vi "Commit DAQ Tags.vi"(8 "error in (no error)":errorcluster, 11 "DAQ State in":T1) -> (0 "error out":errorcluster, 3 "DAQ State out":T1)   [LabVIEW 2018, in "DAQ.lvlib"]
uses:
  DAQ.lvlib
  Acquisition/Hardware Configuration.ctl
  Acquisition/Task Cluster.ctl
  Tag VIs/Tag FGV Operation Enum.ctl
  Shared Variables/Dynamic Shared Variables.lvlib
  <resource>/objmgr/daqmx.rc
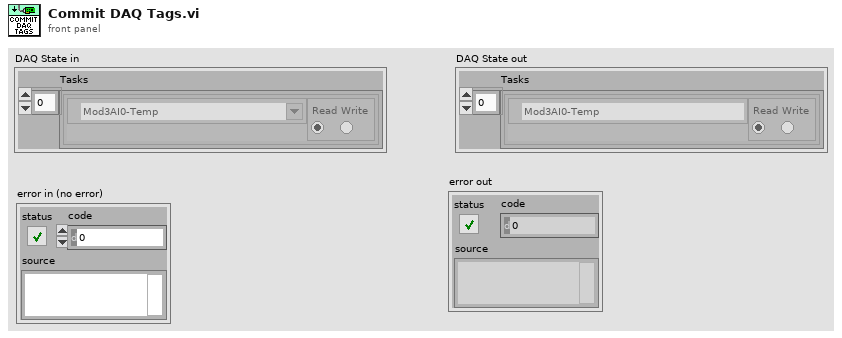
[diagram p1: front panel]
types:
  T1 = typedef "DAQ.lvlib/Hardware Configuration.ctl" = cluster{"Tasks":T2[]}
  T2 = typedef "Task Cluster.ctl" = cluster{"DAQmx Task":refnum<k21>, "Read-Write Radio":enum32{"Read", "Write"}}
  T3 = typedef "Tag FGV Operation Enum.ctl" = enum16{"Init", "Set Notification Queue", "Create Tag", "Commit", "Write Tag (Numeric)", "Write Tag (Boolean)", "Read All Tags", "Read One Tag", "Delete Tag Category", "Set Alarm Parameters (Numeric)", "Set Alarm Parameters (Boolean)", "Enable All Alarms", "Disable All Alarms", "Delete All Tags", "Read Alarms", "Ack Alarm"}
  T4 = enum32{"u32BitField", "bool", "double", "string", "int8", "uint8", "int16", "uint16", "int32", "uint32", "int64", "uint64", "single", "double waveform", "int16 waveform", "array of boolean", "array of int8", "array of uint8", "array of int16", "array of uint16", "array of int32", "array of uint32", "array of int64", "array of uint64", "array of single", "array of double", "array of double waveform", "array of int16 waveform", "array of string", "variant", "timestamp", "fixed point", "custom"}
  T5 = cluster{"enable? (F)":bool, "name":string, "alarm type":enum16{"HI_HI", "HI", "LO", "LO_LO"}, "level/change":dbl, "deadband/time":dbl, "priority":u32, "ack type":enum16{"Auto", "User", "None", "Each Occurrence"}, "area":string, "description":string, "log? (T)":bool}
  T6 = enum16{"Auto", "User", "None", "Each Occurrence"}
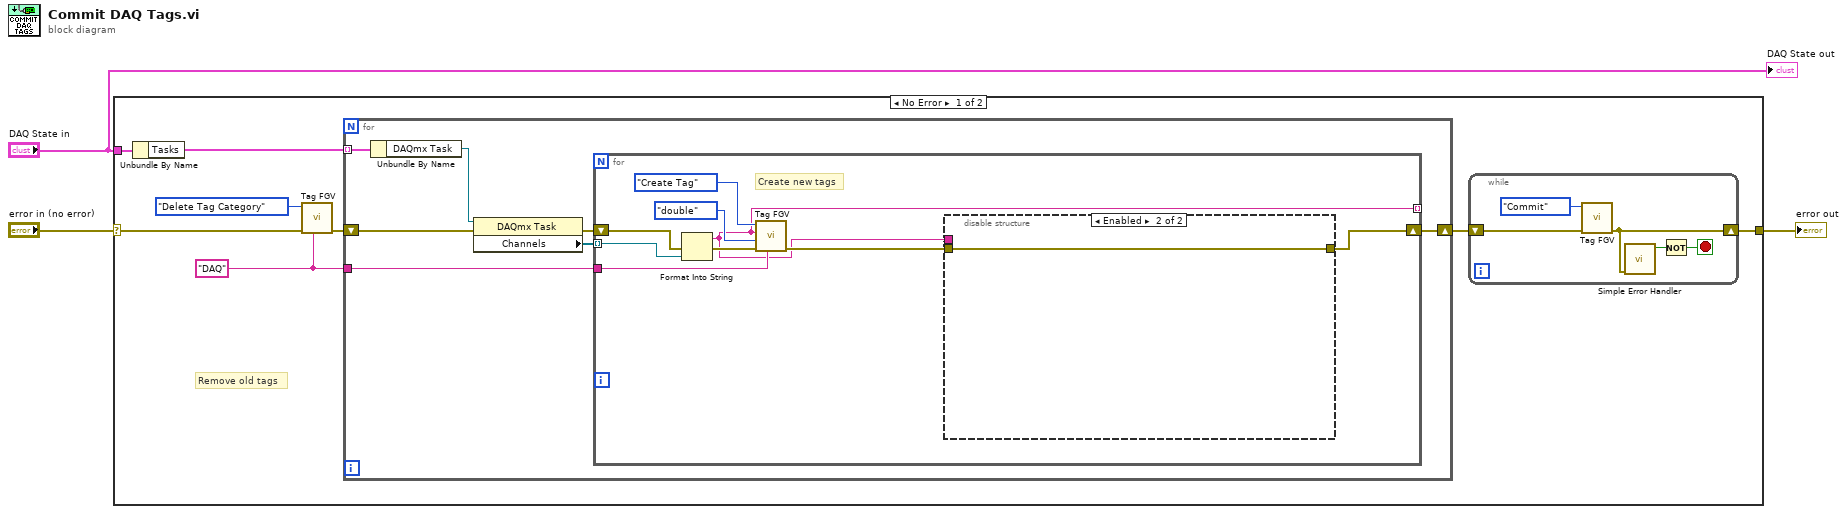
[diagram p0: block diagram]
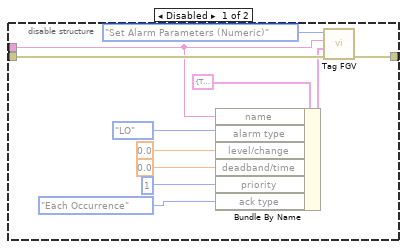
[diagram p2: hidden frame]
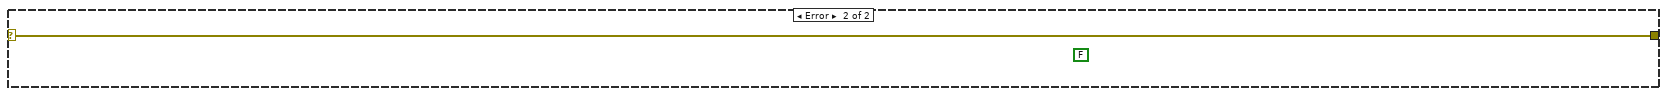
[diagram p3: hidden frame]
diagram:
  n1 = case shown="No Error" "error in (no error)" {
    selector: "error in (no error)" -> [w8 w45]
    tunnel: "DAQ State in" -> [w10 _]
    tunnel: [w4 w45] -> w1
    frame No Error {
      w6 = "DAQ" ("Tag Category")
      # "Remove old tags"
      n2 = Unbundle By Name(w10) -> ("Tasks"=w11:T2[])
      n3 = call "Tag FGV.vi"("Tag Category"=w6, "error in (no error)"=w8, "Operation"=Tag_FGV_Operation_Enum."Delete Tag Category") -> ("error out"=w7:errorcluster)  [unwired: 3 in, 5 out]
      n4 = for {
        tunnel: w11 -> [w23] mode=indexing
        shift-right: [w18] -> w5
        shift-left: w7 -> [w22]
        tunnel: w6 -> [w19]
        n5 = Unbundle By Name(w23) -> ("DAQmx Task"=w21:refnum<k21>)
        n6 = property class="DAQmx Task"(reference=w21, error in=w22) -> (error out=w17:errorcluster, "Channels"=w20:refnum<k21>[])  [unwired: 1 out]
        n7 = for {
          tunnel: w20 -> [w31] mode=indexing
          shift-right: [w25] -> w18
          shift-left: w17 -> [w30]
          tunnel: w19 -> [w27]
          tunnel: [w24] -> _ mode=indexing
          # "Create new tags"
          n8 = Format Into String(error in=w30, w31) -> (resulting string=w24:string, error out=w32:errorcluster)  [unwired: 2 in]
          n9 = call "Tag FGV.vi"("Tag Category"=w27, "error in (no error)"=w32, "Data"=T4."double" ("data type"), "Tag Name"=w24, "Operation"=Tag_FGV_Operation_Enum."Create Tag") -> ("error out"=w26:errorcluster)  [unwired: 1 in, 5 out]
          n10 = disable-structure shown="Enabled" {
            disable-tunnel: w26 -> [w42 w44]
            disable-tunnel: [w41 w44] -> w25
            disable-tunnel: w24 -> [w39 _]
            frame Disabled {
              n11 = Bundle By Name(cluster=T5 {"enable? (F)"=TRUE, "name"="HiHi", "alarm type"=enum."HI_HI", "level/change"=50.0, "deadband/time"=1.0, "priority"=1, "ack type"=enum."Each Occurrence", "area"="", "description"="", "log? (T)"=TRUE} ("numeric alarm settings"), "name"=w39, "alarm type"=enum16{"HI_HI", "HI", "LO", "LO_LO"}."LO", "level/change"=0.0, "deadband/time"=0.0, "priority"=u32 1, "ack type"=T6."Each Occurrence") -> (w33:T5)
              n12 = call "Tag FGV.vi"("error in (no error)"=w42, "Data"=w33, "Tag Name"=w39, "Operation"=Tag_FGV_Operation_Enum."Set Alarm Parameters (Numeric)") -> ("error out"=w41:errorcluster)  [unwired: 2 in, 5 out]
            }
            frame Enabled {
            }
          }
        }
      }
      n13 = while {
        shift-right: [w14] -> w4
        shift-left: w5 -> [w15]
        stop <- w12 stop-if-true
        n14 = call "Tag FGV.vi"("error in (no error)"=w15, "Operation"=Tag_FGV_Operation_Enum."Commit") -> ("error out"=w14:errorcluster)  [unwired: 4 in, 5 out]
        n15 = call <vilib>:"Simple Error Handler.vi"("error in (no error)"=w14) -> ("error?"=w13:bool)  [unwired: 4 in, 4 out]
        n16 = Not(x=w13) -> (.not. x?=w12:bool)
      }
    }
    frame Error {
      (unwired) FALSE
    }
  }
  "error out" <- w1
  "DAQ State out" <- "DAQ State in"
